vi "CODcr 随机数出数.vi"(4 "公式":cluster{"X^2":dbl, "X":dbl, "B":dbl}, 5 "测试模式":enum16{"水样测试", "零点核查", "跨度核查"}(ring), 8 "信号值原始值":dbl, 9 "原始值":dbl) -> (2 "信号值":dbl, 3 "取值输出":dbl)   [LabVIEW 2016]
uses:
  Holding Var.vi
  Process var.vi
  random number/random number.lvlib
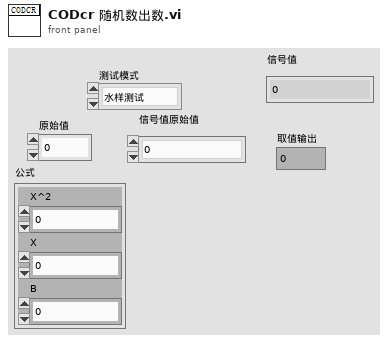
[diagram p1: front panel]
types:
  T1 = cluster{"水样参数输出":cluster{"mean":dbl, "变异系数":dbl, "随机数？":bool}, "零点参数输出":cluster{"mean":dbl, "变异系数":dbl, "随机数？":bool}, "跨度参数输出":cluster{"mean":dbl, "变异系数":dbl, "随机数？":bool}}
  T2 = cluster{"水样测试":cluster{"参数输入":cluster{"采样模式":enum16{"自动采样", "手动采样"}, "采样点数":i32, "变异系数设定值":dbl, "重新取值百分比":dbl, "偏差模式":enum16{"相对偏差", "绝对偏差"}, "相对偏差百分比":dbl, "绝对偏差值":dbl}, "采样值":dbl[], "启用":bool}, "零点核查":cluster{"参数输入":cluster{"采样模式":enum16{"自动采样", "手动采样"}, "采样点数":i32, "变异系数设定值":dbl, "重新取值百分比":dbl, "偏差模式":enum16{"相对偏差", "绝对偏差"}, "相对偏差百分比":dbl, "绝对偏差值":dbl}, "采样值":dbl[], "启用":bool}, "跨度核查":cluster{"参数输入":cluster{"采样模式":enum16{"自动采样", "手动采样"}, "采样点数":i32, "变异系数设定值":dbl, "重新取值百分比":dbl, "偏差模式":enum16{"相对偏差", "绝对偏差"}, "相对偏差百分比":dbl, "绝对偏差值":dbl}, "采样值":dbl[], "启用":bool}}
  T3 = cluster{"采样模式":enum16{"自动采样", "手动采样"}, "采样点数":i32, "变异系数设定值":dbl, "重新取值百分比":dbl, "偏差模式":enum16{"相对偏差", "绝对偏差"}, "相对偏差百分比":dbl, "绝对偏差值":dbl}
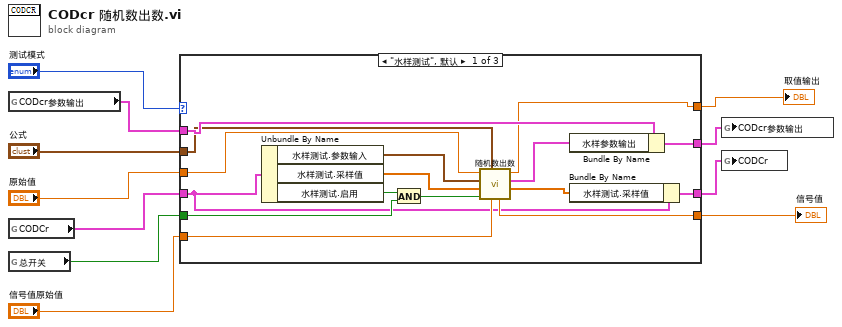
[diagram p0: block diagram]
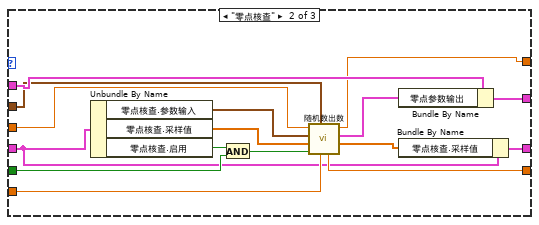
[diagram p2: hidden frame]
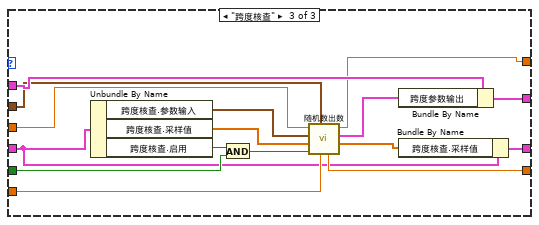
[diagram p3: hidden frame]
diagram:
  n1 = global read "Process var.vi" "CODcr参数输出"() -> (w10:T1)
  n2 = global read "Holding Var.vi" "CODCr"() -> (w11:T2)
  n3 = global read "Holding Var.vi" "总开关"() -> (w5:bool)
  n4 = case shown="\"水样测试\", 默认" "测试模式" {
    tunnel: w11 -> [w14 w30 w46]
    tunnel: w10 -> [w25 w41 w57]
    tunnel: [w23 w39 w55] -> w9
    tunnel: "原始值" -> [w22 w38 w54]
    tunnel: [w21 w37 w53] -> w6
    tunnel: w5 -> [w20 w36 w52]
    tunnel: "公式" -> [w17 w33 w49]
    tunnel: "信号值原始值" -> [w16 w32 w48]
    tunnel: [w15 w31 w47] -> w2
    tunnel: [w13 w28 w44] -> w1
    frame "水样测试", Default {
      n5 = Unbundle By Name(w14) -> ("水样测试.参数输入"=w27:T3, "水样测试.采样值"=w26:dbl[], "水样测试.启用"=w19:bool)
      n6 = And(x=w19, y=w20) -> (x .and. y?=w18:bool)
      n7 = call "随机数出数.vi"("信号值原始值"=w16, "公式"=w17, "启用"=w18, "采样值"=w26, "参数输入"=w27, "监测值原始值"=w22) -> ("采样值输出"=w12:dbl[], "参数输出"=w24:cluster{"mean":dbl, "变异系数":dbl, "随机数？":bool}, "取值输出"=w21:dbl, "信号值"=w15:dbl)  [unwired: 2 in]
      n8 = Bundle By Name(cluster=w25, "水样参数输出"=w24) -> (w23:T1)
      n9 = Bundle By Name(cluster=w14, "水样测试.采样值"=w12) -> (w13:T2)
    }
    frame "零点核查" {
      n10 = Unbundle By Name(w30) -> ("零点核查.参数输入"=w43:T3, "零点核查.采样值"=w42:dbl[], "零点核查.启用"=w35:bool)
      n11 = And(x=w35, y=w36) -> (x .and. y?=w34:bool)
      n12 = call "随机数出数.vi"("信号值原始值"=w32, "公式"=w33, "启用"=w34, "采样值"=w42, "参数输入"=w43, "监测值原始值"=w38) -> ("采样值输出"=w29:dbl[], "参数输出"=w40:cluster{"mean":dbl, "变异系数":dbl, "随机数？":bool}, "取值输出"=w37:dbl, "信号值"=w31:dbl)  [unwired: 2 in]
      n13 = Bundle By Name(cluster=w41, "零点参数输出"=w40) -> (w39:T1)
      n14 = Bundle By Name(cluster=w30, "零点核查.采样值"=w29) -> (w28:T2)
    }
    frame "跨度核查" {
      n15 = Unbundle By Name(w46) -> ("跨度核查.参数输入"=w59:T3, "跨度核查.采样值"=w58:dbl[], "跨度核查.启用"=w51:bool)
      n16 = And(x=w51, y=w52) -> (x .and. y?=w50:bool)
      n17 = call "随机数出数.vi"("信号值原始值"=w48, "公式"=w49, "启用"=w50, "采样值"=w58, "参数输入"=w59, "监测值原始值"=w54) -> ("采样值输出"=w45:dbl[], "参数输出"=w56:cluster{"mean":dbl, "变异系数":dbl, "随机数？":bool}, "取值输出"=w53:dbl, "信号值"=w47:dbl)  [unwired: 2 in]
      n18 = Bundle By Name(cluster=w57, "跨度参数输出"=w56) -> (w55:T1)
      n19 = Bundle By Name(cluster=w46, "跨度核查.采样值"=w45) -> (w44:T2)
    }
  }
  "取值输出" <- w6
  "信号值" <- w2
  n20 = global write "Process var.vi" "CODcr参数输出"(w9) -> ()
  n21 = global write "Holding Var.vi" "CODCr"(w1) -> ()
